vi "Remove Bad Points.vi"(8 "error in (no error)":errorcluster, 10 "Database Trace In":T1(array[cluster]), 11 "Database Viewer":refnum<class "Database Viewer.lvclass">) -> (0 "error out":errorcluster, 2 "Database Trace Out":T1(array[cluster]), 3 "Database Viewer out":refnum<class "Database Viewer.lvclass">)   [LabVIEW 2019, in "Database Viewer.lvclass"]
uses:
  Database Viewer.lvclass
  <userlib>/_OpenG.lib/array/array.llb/Search 1D Array (Variant)__ogtk.vi
  <userlib>/_OpenG.lib/array/array.llb/Delete Elements from 1D Array (DBL)__ogtk.vi
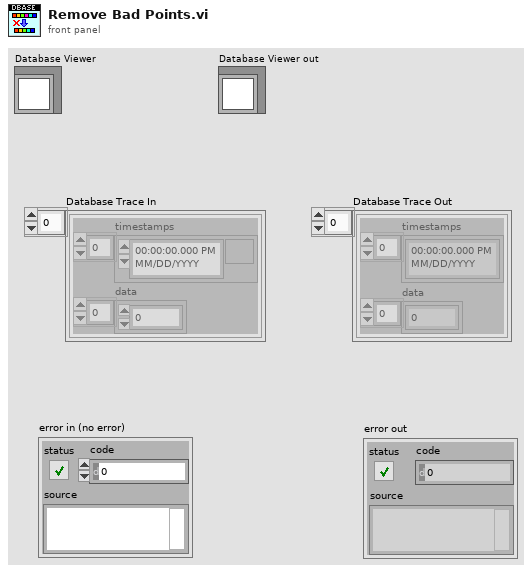
[diagram p1: front panel]
types:
  T1 = cluster{"timestamps":timestamp[], "data":dbl[]}[]
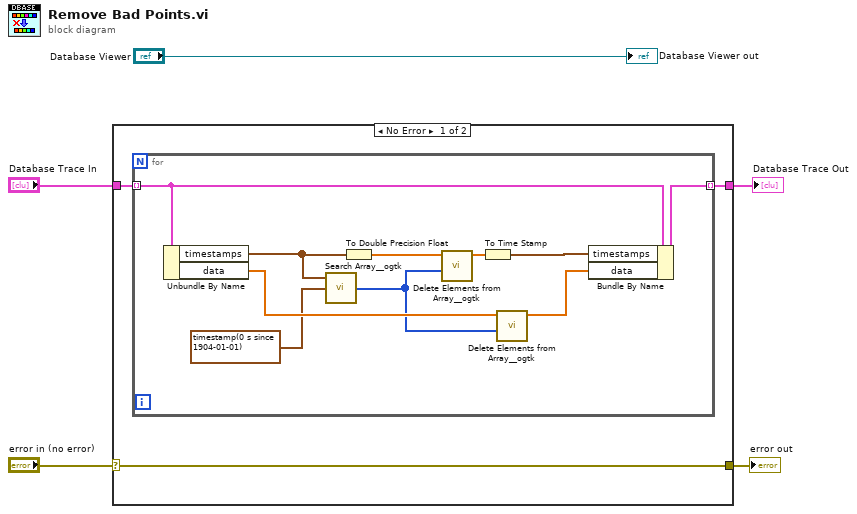
[diagram p0: block diagram]
diagram:
  n1 = case shown="No Error" "error in (no error)" {
    selector: "error in (no error)" -> [w6 w20]
    tunnel: "Database Trace In" -> [w8 w19]
    tunnel: [w7 w19] -> w4
    tunnel: [w6 w20] -> w2
    frame No Error {
      n2 = for {
        tunnel: w8 -> [w18] mode=indexing
        tunnel: [w17] -> w7 mode=indexing
        n3 = Unbundle By Name(w18) -> ("timestamps"=w9:timestamp[], "data"=w15:dbl[])
        n4 = call-poly <userlib>:"Search Array__ogtk.vi"("Array"=w9, "Element Data"=timestamp(0 s since 1904-01-01) ("Timestamp")) -> ("Indices of Elements"=w11:i32[])  [unwired: 7 in]
        n5 = To Double Precision Float(number=w9) -> (double precision float=w14:dbl[])
        n6 = call-poly <userlib>:"Delete Elements from Array__ogtk.vi"("indices"=w11, "array"=w14) -> ("array w/ subset deleted"=w13:dbl[])  [unwired: 8 in, 1 out]
        n7 = To Time Stamp(1:w13) -> (0:w12:timestamp[])
        n8 = call-poly <userlib>:"Delete Elements from Array__ogtk.vi"("indices"=w11, "array"=w15) -> ("array w/ subset deleted"=w16:dbl[])  [unwired: 8 in, 1 out]
        n9 = Bundle By Name(cluster=w18, "timestamps"=w12, "data"=w16) -> (w17:cluster{"timestamps":timestamp[], "data":dbl[]})
      }
    }
    frame Error {
    }
  }
  "Database Trace Out" <- w4
  "error out" <- w2
  "Database Viewer out" <- "Database Viewer"
